vi "Main UI.vi"(8 "error in (no error)":errorcluster, 11 "Timer Demo App in":refnum<class "Timer Demo App.lvclass">) -> (0 "error out":errorcluster, 3 "Timer Demo App out":refnum<class "Timer Demo App.lvclass">)   [LabVIEW 2020, in "Timer Demo.lvlib" / "Timer Demo App.lvclass"]
uses:
  Timer Demo App.lvclass
  Timer Action Response.ctl
  Timer Demo.lvlib
  Timer Status Response.ctl
  lv-http-server/HTTP Server/Server/Server.lvclass
  lv-http-server/HTTP Server/RequestTraceLog/RequestTraceLog.lvclass
  lv-http-server/HTTP Server/Processing Step.ctl
  lv-http-server/HTTP Server/HTTP Server.lvlib
  lv-http-server/HTTP Server/Trace Item.ctl
  lv-http-util/HTTP Utils/Method.ctl
  lv-http-util/HTTP Utils/HTTP Utils.lvlib
  lv-http-server/HTTP Server/Trace Log.ctl
panel:
  in  "Refresh Traces":bool
  out "Traces":T1[](array[typedef])=[{"Items"=[{"Duration"=0.00019280000014987309, "Step"=enum."Connection", "Class"="", "Info"="Start Request Parsing", "Status"=FALSE, "Code"=0, "Time"=3234.2736639}, {"Duration"=104.21120999999994, "Step"=enum."Connection", "Class"="", "Info"="Request Initialized", "Status"=TRUE, "Code"=66, "Time"=3338.4848739}, {"Duration"=0.0007422999997288571, "Step"=enum."Connection", "Class"="HTTP Utils.lvlib:Response.lvclass", "Info"="Completed", "Status"=TRUE, "Code"=66, "Time"=3338.4856161999996}], "Client"="tcp://DAB-2020SP1x86.ni.corp.natinst.com:52788", "Target"="", "Response Type"="", "Processing"=0.0007728000000497559, "Status"=200, "Method"=enum."GET", "Content Type"="", "Request Headers"=[], "Parsing"=3338.4848739, "Waiting"=-3234.2736639, "Identity"="", "Loaded"=FALSE, "Created"=FALSE, "Destroyed"=FALSE, "Response Headers"=[], "Created"=0.0, "Expires"=0.0, "Roles"=[], "Sending"=0.0}, {"Items"=[{"Duration"=0.006463199999870994, "Step"=enum."Connection", "Class"="", "Info"="Start Request Parsing", "Status"=FALSE, "Code"=0, "Time"=3459.3199179}, {"Duration"=0.008297200000015437, "Step"=enum."Connection", "Class"="", "Info"="Request Initialized", "Status"=TRUE, "Code"=66, "Time"=3459.3282151}, {"Duration"=0.0001554000000396627, "Step"=enum."Connection", "Class"="HTTP Utils.lvlib:Response.lvclass", "Info"="Completed", "Status"=TRUE, "Code"=66, "Time"=3459.3283705}], "Client"="tcp://DAB-2020SP1x86.ni.corp.natinst.com:52995", "Target"="", "Response Type"="", "Processing"=0.00019930000007661874, "Status"=200, "Method"=enum."GET", "Content Type"="", "Request Headers"=[], "Parsing"=3459.3282151, "Waiting"=-3459.3199179, "Identity"="", "Loaded"=FALSE, "Created"=FALSE, "Destroyed"=FALSE, "Response Headers"=[], "Created"=0.0, "Expires"=0.0, "Roles"=[], "Sending"=0.0}] {"Sending" format="%_6f"; "Expires" format="%<%X %x>T"; "Created" format="%<%X %x>T"; "Waiting" format="%_6f"; "Parsing" format="%_6f"; "Processing" format="%_6f"; "Items"."Time" format="%.6f"; "Items"."Duration" format="%.6f"}
  out "Running":bool
  out "Elapsed":dbl
  # "Start the timer with\nhttp://localhost:36987/timer/action?op=start"
  # "Trying to start a timer when it's already started or pause a timer when it's not started will result in an error response being generated."
  # "View the timer value at\nhttp://localhost:36987/timer/status"
  # "Pause the timer with\nhttp://localhost:36987/timer/action?op=pause"
  # "Reset the timer with\nhttp://localhost:36987/timer/action?op=reset"
  # "Request"
  # "Response"
  # "Session"
  # "Auth"
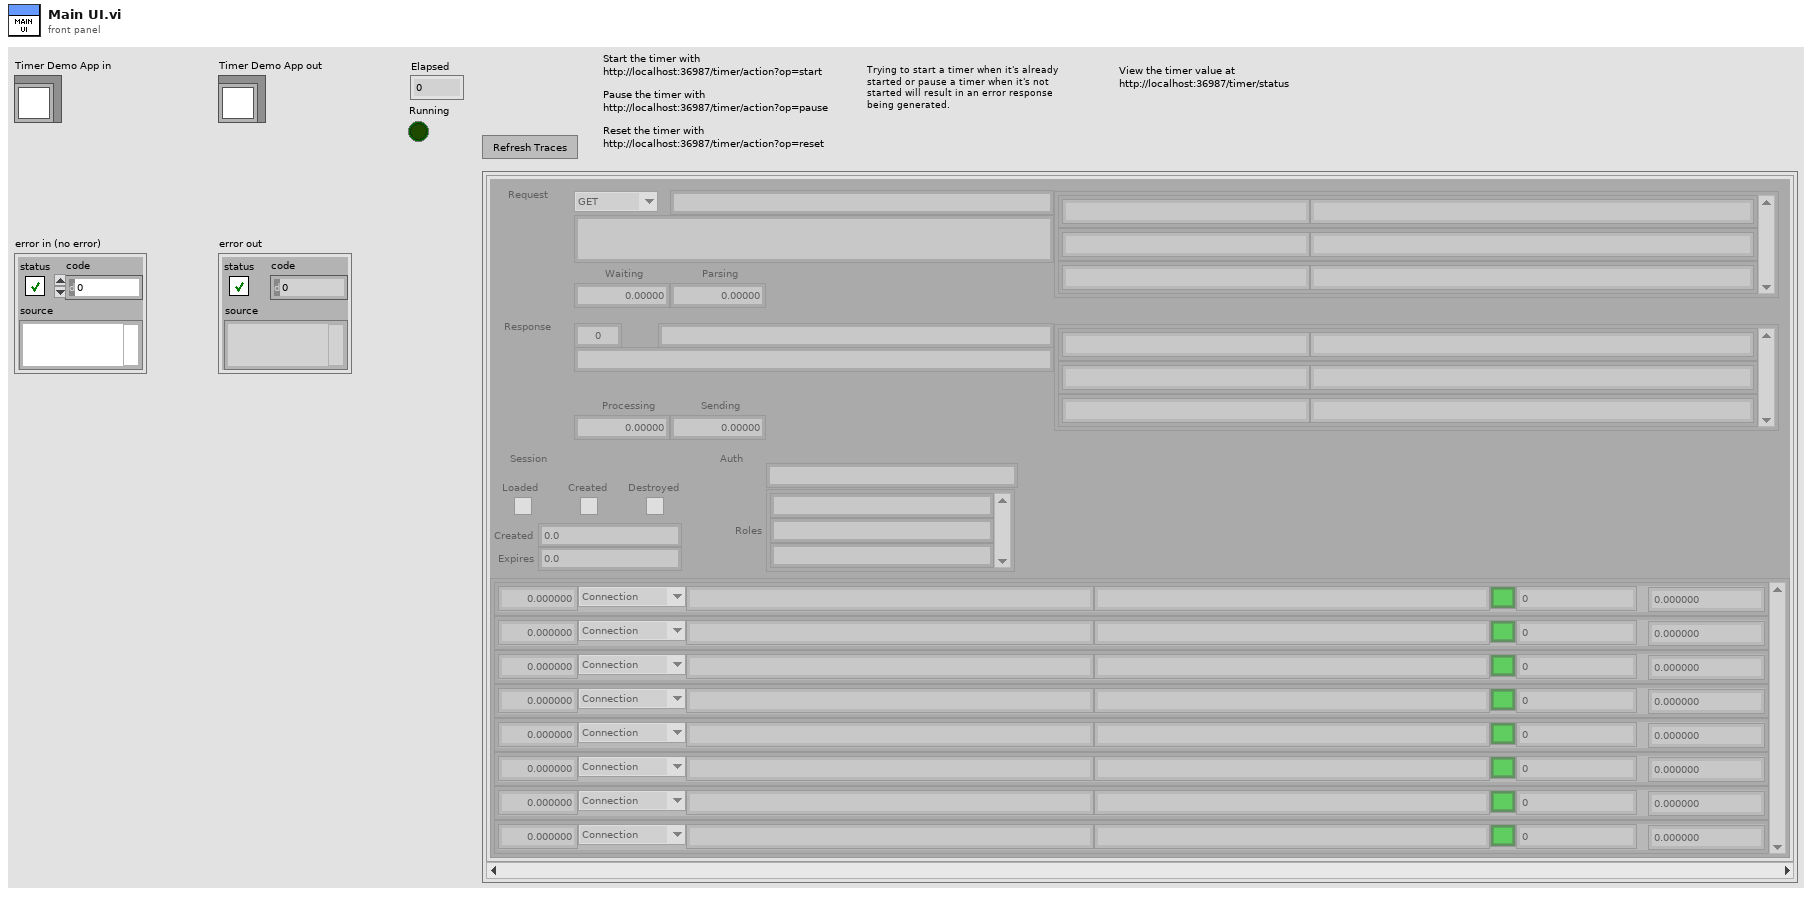
[diagram p1: front panel]
types:
  T1 = typedef "HTTP Server.lvlib/Trace Log.ctl" = cluster{"Items":T2[], "Client":string, "Target":string, "Response Type":string, "Processing":dbl, "Status":u16, "Method":T4, "Content Type":string, "Request Headers":cluster{"Name":string, "Value":string}[], "Parsing":dbl, "Waiting":dbl, "Identity":string, "Loaded":bool, "Created":bool, "Destroyed":bool, "Response Headers":cluster{"Name":string, "Value":string}[], "Created":dbl, "Expires":dbl, "Roles":string[], "Sending":dbl}
  T2 = typedef "HTTP Server.lvlib/Trace Item.ctl" = cluster{"Duration":dbl, "Step":T3, "Class":string, "Info":string, "Status":bool, "Code":i32, "Time":dbl}
  T3 = typedef "HTTP Server.lvlib/Processing Step.ctl" = enum16{"Connection", "Request", "Routing", "Controller Init", "Controller", "Response", "Complete", "Exception"}
  T4 = typedef "HTTP Utils.lvlib/Method.ctl" = enum16{"GET", "HEAD", "POST", "PUT", "DELETE", "CONNECT", "OPTIONS", "TRACE", "PATCH"}
  T5 = typedef "Timer Demo.lvlib/Timer Action Response.ctl" = cluster{"Error":errorcluster}
  T6 = typedef "Timer Demo.lvlib/Timer Status Response.ctl" = cluster{"Elapsed":dbl, "Running":bool}
  T7 = typedef "Timer Demo.lvlib/Timer Action.ctl" = enum16{"start", "pause", "reset"}
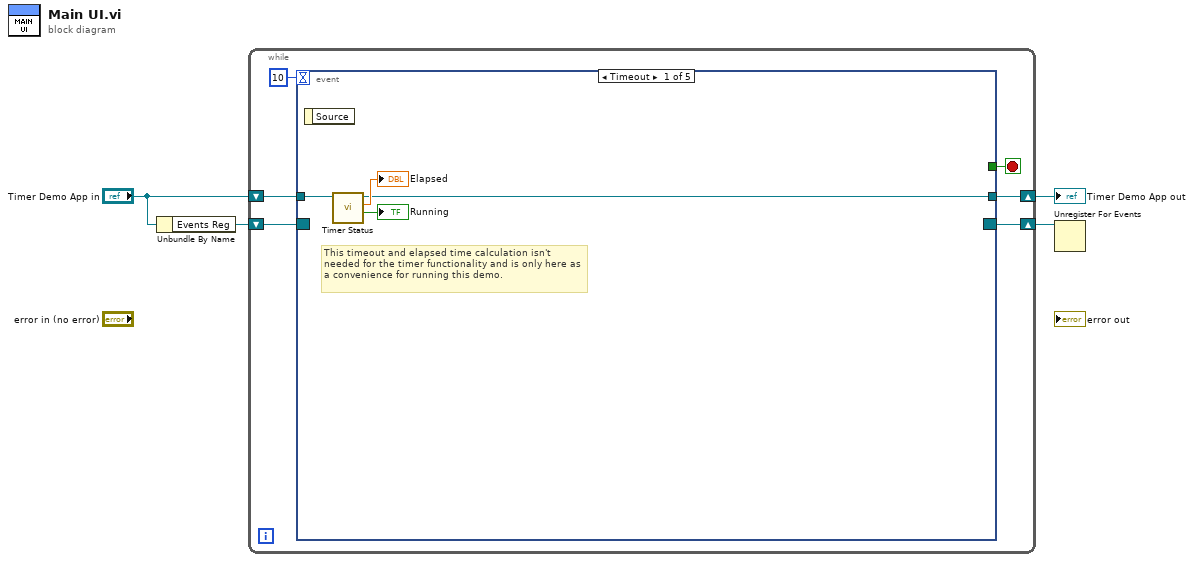
[diagram p0: block diagram]
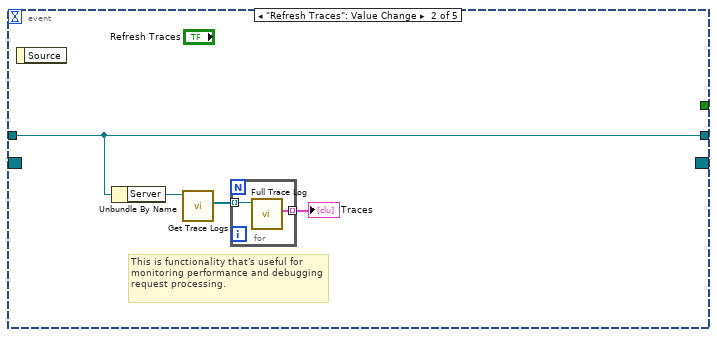
[diagram p2: hidden frame]
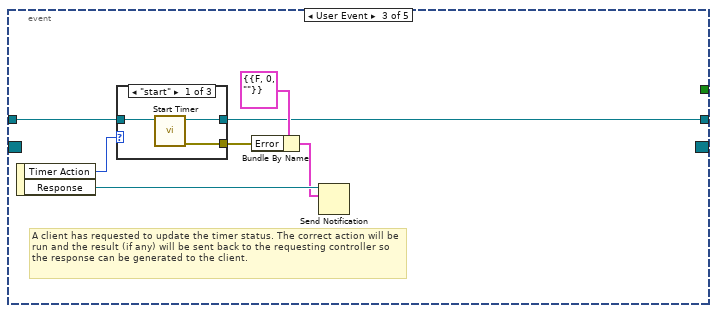
[diagram p3: hidden frame]
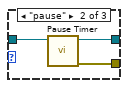
[diagram p4: hidden frame]
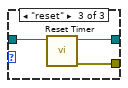
[diagram p5: hidden frame]
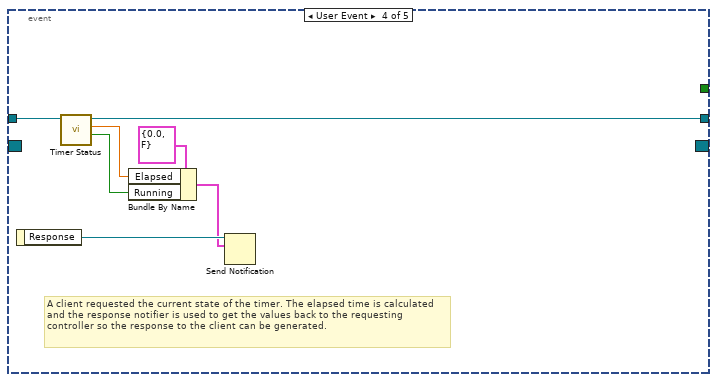
[diagram p6: hidden frame]
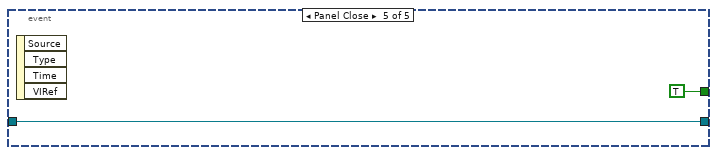
[diagram p7: hidden frame]
diagram:
  n1 = Unbundle By Name("Timer Demo App in") -> ("Events Reg"=w3:refnum<event-registration>)
  n2 = while {
    shift-right: [w8] -> w1
    shift-left: w3 -> [w9]
    shift-right: [w7] -> w2
    shift-left: "Timer Demo App in" -> [w10]
    stop <- w6 stop-if-true
    n3 = event shown="[0] Timeout" {
      selector: w9 -> [_ _ _ _ _]
      dyn-events: [_ _ _ _ _] -> w8
      timeout: 10 -> [_ _ _ _ _]
      tunnel: w10 -> [w14 w17 w27 w41 w45]
      tunnel: [w12 w17 w22 w40 w45] -> w7
      tunnel: [_ _ _ _ TRUE] -> w6
      event Timeout {
        # "This timeout and elapsed time calculation isn't needed for the timer functionality and is only here as a convenience for running this demo."
        n4 = event-data() -> ()  [unwired: 1 in, 1 out]
        n5 = call "Timer Status.vi"("Timer Demo App in"=w14) -> ("Running"=→"Running":bool, "Elapsed"=→"Elapsed":dbl, "Timer Demo App out"=w12:refnum<class "Timer Demo App.lvclass">)  [unwired: 7 in, 1 out]
      }
      event "Refresh Traces": Value Change {
        # "This is functionality that's useful for monitoring performance and debugging request processing."
        n6 = event-data() -> ()  [unwired: 1 in, 1 out]
        n7 = Unbundle By Name(w17) -> ("Server"=w16:refnum<class "Server.lvclass">)
        n8 = call "Get Trace Logs.vi"("Server in"=w16) -> ("Trace Logs"=w18:refnum<class "RequestTraceLog.lvclass">[])  [unwired: 8 in, 2 out]
        n9 = for {
          tunnel: w18 -> [w20] mode=indexing
          tunnel: [w19] -> w15 mode=indexing
          n10 = call "Full Trace Log.vi"("RequestTraceLog in"=w20) -> ("Trace Log"=w19:T1)  [unwired: 8 in, 2 out]
        }
        "Traces" <- w15
      }
      event User Event {
        # "A client has requested to update the timer status. The correct action will be run and the result (if any) will be sent back to the requesting controller so the response can be generated to the client."
        n11 = event-data() -> ("Timer Action"=w26:T7, "Response"=w25:refnum<notifier>)  [unwired: 1 in]
        n12 = case shown="\"start\"" w26 {
          tunnel: w27 -> [w30 w33 w36]
          tunnel: [w29 w32 w35] -> w22
          tunnel: [w28 w31 w34] -> w21
          frame "start" {
            n13 = call "Start Timer.vi"("Timer Demo App in"=w30) -> ("error out"=w28:errorcluster, "Timer Demo App out"=w29:refnum<class "Timer Demo App.lvclass">)  [unwired: 9 in]
          }
          frame "pause" {
            n14 = call "Pause Timer.vi"("Timer Demo App in"=w33) -> ("error out"=w31:errorcluster, "Timer Demo App out"=w32:refnum<class "Timer Demo App.lvclass">)  [unwired: 9 in]
          }
          frame "reset" {
            n15 = call "Reset Timer.vi"("Timer Demo App in"=w36) -> ("error out"=w34:errorcluster, "Timer Demo App out"=w35:refnum<class "Timer Demo App.lvclass">)  [unwired: 9 in]
          }
        }
        n16 = Bundle By Name(cluster=T5 {"Error"={"status"=FALSE, "code"=0, "source"=""}} ("notification"), "Error"=w21) -> (w23:T5)
        n17 = Send Notification(notification=w23, notifier=w25) -> ()  [unwired: 1 in, 2 out]
      }
      event User Event {
        # "A client requested the current state of the timer. The elapsed time is calculated and the response notifier is used to get the values back to the requesting controller so the response to the client can be generated."
        n18 = event-data() -> ("Response"=w43:refnum<notifier>)  [unwired: 1 in]
        n19 = call "Timer Status.vi"("Timer Demo App in"=w41) -> ("Running"=w37:bool, "Elapsed"=w38:dbl, "Timer Demo App out"=w40:refnum<class "Timer Demo App.lvclass">)  [unwired: 7 in, 1 out]
        n20 = Bundle By Name(cluster=T6 {"Elapsed"=0.0, "Running"=FALSE} ("notification"), "Elapsed"=w38, "Running"=w37) -> (w39:T6)
        n21 = Send Notification(notification=w39, notifier=w43) -> ()  [unwired: 1 in, 2 out]
      }
      event Panel Close {
        n22 = event-data() -> ()  [unwired: 1 in, 4 out]
      }
    }
  }
  "Timer Demo App out" <- w2
  n23 = Unregister For Events(event registration refnum=w1) -> ()  [unwired: 1 in, 1 out]
